vi "Msg.vi"(7 "jettl in":refnum<class "jettl.lvclass">, 11 "Create Queue Msg Strategy in":refnum<class "Create Queue Msg Strategy.lvclass">) -> (5 "jettl out":refnum<class "jettl.lvclass">)   [LabVIEW 2021, in "Create Queue Msg Strategy.lvlib" / "Create Queue Msg Strategy.lvclass"]
uses:
  Create Queue Msg Strategy.lvclass
  jettl/jettl/jettl.lvclass
  Create Queue/Create Queue.lvclass
  Create Queue Msg Strategy.lvclass/Create Queue Msg Strategy.ctl
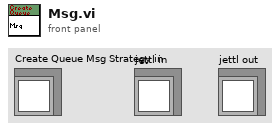
[diagram p1: front panel]
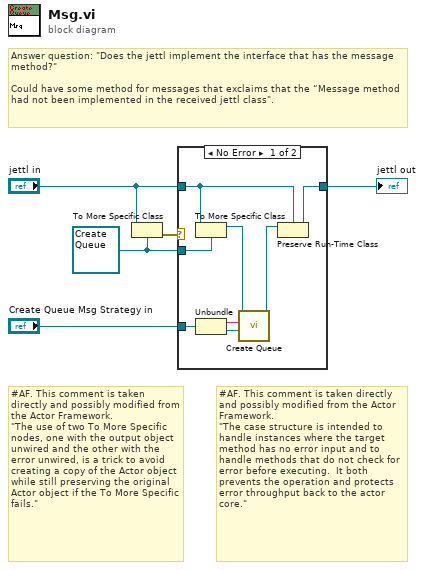
[diagram p0: block diagram]
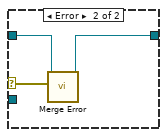
[diagram p2: hidden frame]
diagram:
  w4 = refnum<class "Create Queue.lvclass"> refnum ("Create.lvlib:Create.lvclass")
  # "#AF. This comment is taken directly and possibly modified from the Actor Framework.\n\"The use of two To More Specific nodes, one with the output object unwired and the other with the error unwired, is a trick to avoid creating a copy of the Actor object while still preserving the original Actor object if the To More Specific fails.\""
  # "#AF. This comment is taken directly and possibly modified from the Actor Framework.\n\"The case structure is intended to handle instances where the target method has no error input and to handle methods that do not check for error before executing.  It both prevents the operation and protects error throughput back to the actor core.\""
  # "Answer question: \"Does the jettl implement the interface that has the message method?\"\n\nCould have some method for messages that exclaims that the “Message method had not been implemented in the received jettl class\"."
  n1 = To More Specific Class(target class=w4, reference="jettl in") -> (error out=w5:errorcluster)  [unwired: 1 in, 1 out]
  n2 = case shown="No Error" w5 {
    selector: w5 -> [_ w16]
    tunnel: [w8 w14] -> w1
    tunnel: "jettl in" -> [w9 w15]
    tunnel: w4 -> [w13 _]
    tunnel: "Create Queue Msg Strategy in" -> [w12 _]
    frame No Error {
      n3 = To More Specific Class(target class=w13, reference=w9) -> (specific class reference=w7:refnum<class "Create Queue.lvclass">)  [unwired: 1 in, 1 out]
      n4 = Unbundle(w12) -> (w11:string, w10:refnum<class "Queue.lvclass">)
      n5 = call-dynamic "Create Queue.vi"("Queue"=w10, "Self Queue Alias"=w11, "jettl Msg Create Queue in"=w7) -> ("jettl Msg Create Queue out"=w6:refnum<class "Create Queue.lvclass">)  [unwired: 8 in]
      n6 = Preserve Run-Time Class(object in=w6, 2:w9) -> (object out=w8:refnum<class "jettl.lvclass">)  [unwired: 1 in, 1 out]
    }
    frame Error {
      n7 = call-dynamic "Merge Error.vi"("Error"=w16, "Merge Error in"=w15) -> ("Merge Error out"=w14:refnum<class "jettl.lvclass">)  [unwired: 9 in]
    }
  }
  "jettl out" <- w1
